vi "test - click.vi"() -> ()   [LabVIEW 2020]
uses:
  <vilib>/Utility/miscctls.llb/LVPositionTypeDef.ctl
  <vilib>/Utility/miscctls.llb/LVPointTypeDef.ctl
  ui-testing.lvlib
  User32.dll
panel:
  out "Screen Coordinates":T1
  out "PanelCoords 2":T1
  out "PanelCoords":T1
  out "Position":T2
  in  "OK Button":bool
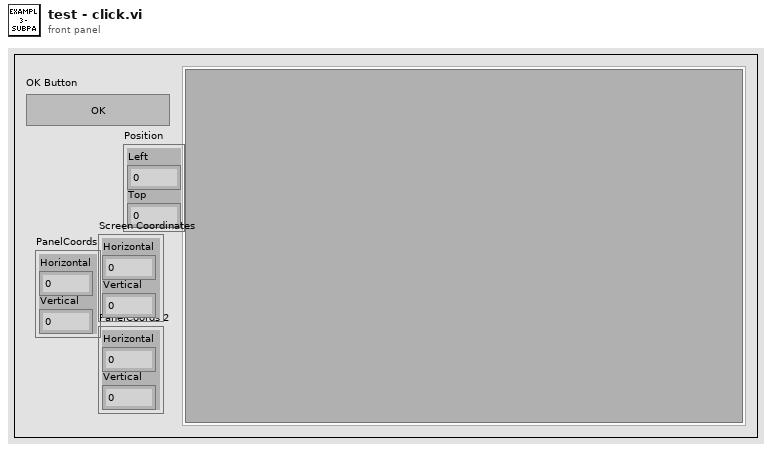
[diagram p1: front panel]
types:
  T1 = typedef "LVPointTypeDef.ctl" = cluster{"Horizontal":i16, "Vertical":i16}
  T2 = typedef "LVPositionTypeDef.ctl" = cluster{"Left":i32, "Top":i32}
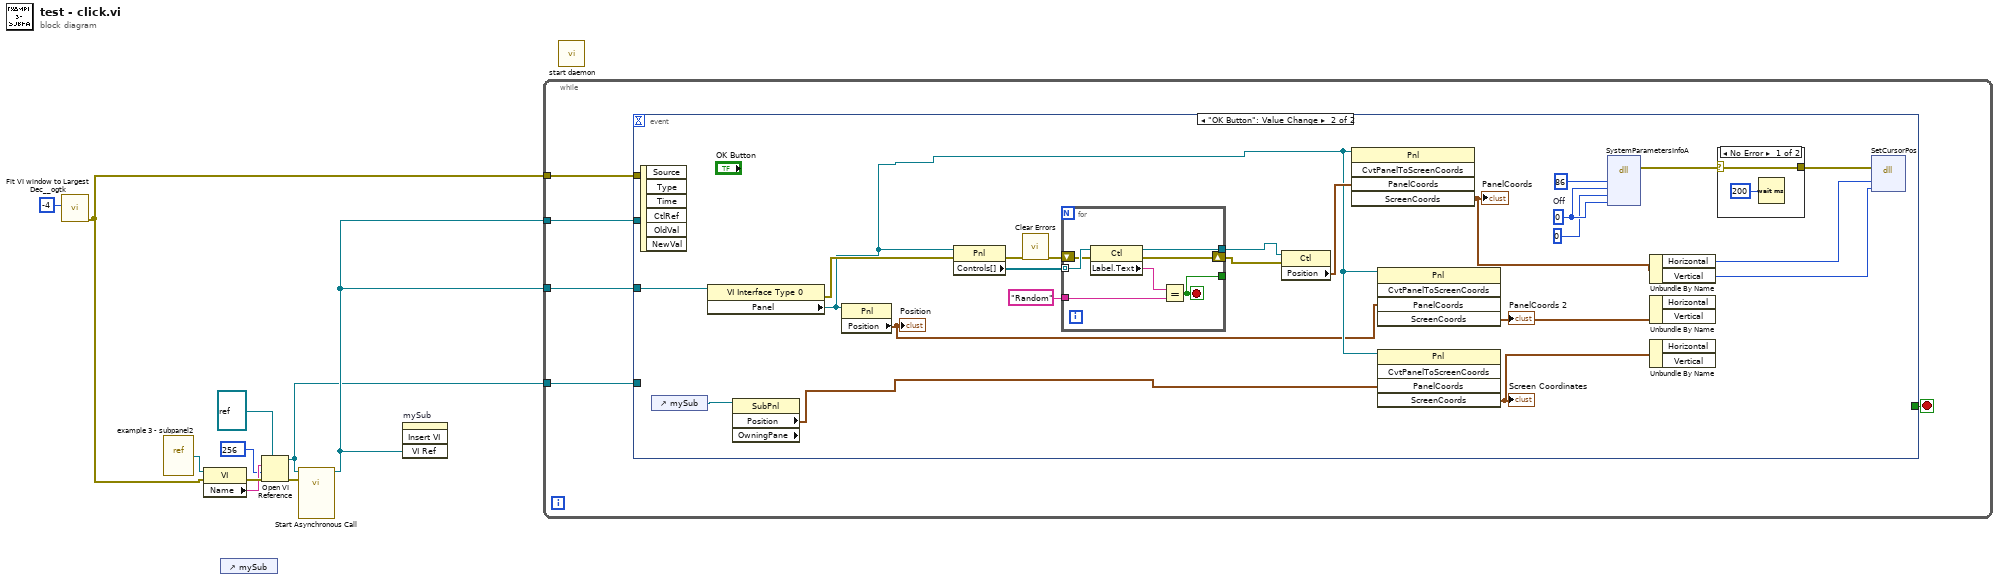
[diagram p0: block diagram]
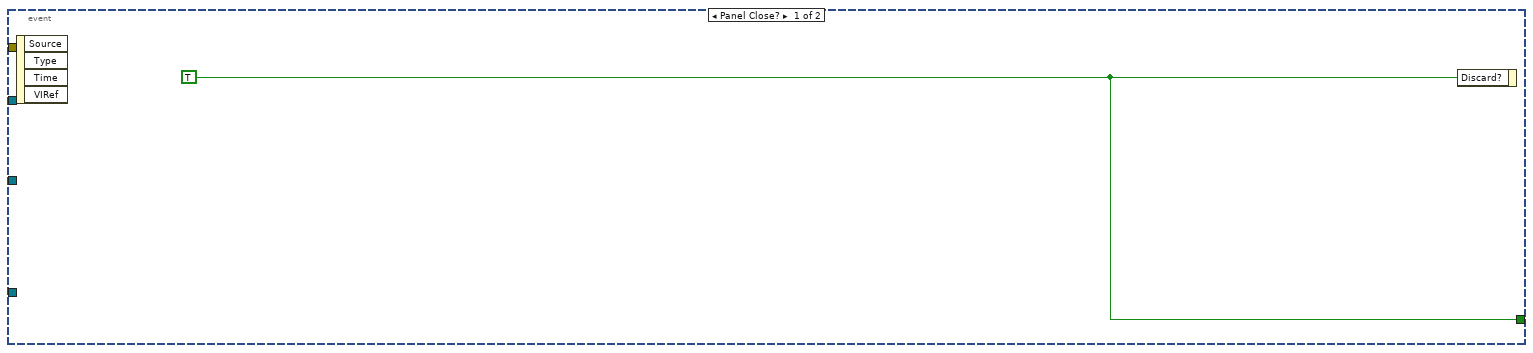
[diagram p2: hidden frame]
diagram:
  n1 = call <userlib>:"Fit VI window to Largest Dec__ogtk.vi"("border spacing (2 px)"=-4) -> ("error out"=w3:errorcluster)  [unwired: 5 in, 1 out]
  n2 = vi-ref "example 3 - subpanel2.vi"() -> (w8:refnum<vi>)
  n3 = property class="VI"(reference=w8, error in=w3) -> (error out=w10:errorcluster, "Name"=w9:string)  [unwired: 1 out]
  n4 = control-ref of="mySub"() -> ()  [unwired: 1 out]
  n5 = Open VI Reference(type specifier VI Refnum (for type only)=refnum<vi> refnum, vi path=w9, options=256 ("call and forget"), error in (no error)=w10) -> (vi reference=w1:refnum<vi>, error out=w7:errorcluster)  [unwired: 2 in]
  n6 = call-by-ref "Start Asynchronous Call"(reference=w1, error in=w7) -> (reference out=w2:refnum<vi>)  [unwired: 12 in, 1 out]
  n7 = invoke on="mySub" class="SubPnl" method="Insert VI"("VI Ref"=w2) -> ()  [unwired: 3 in, 4 out]
  n8 = while {
    tunnel: w3 -> [w14]
    tunnel: w2 -> [w13]
    tunnel: w2 -> [w12]
    tunnel: w1 -> [w11]
    stop <- w15 stop-if-true
    n9 = event shown="[1] \"OK Button\": Value Change" {
      selector: _ -> [_ _]
      dyn-events: _ -> [_ _]
      timeout: _ -> [_ _]
      tunnel: [w16 _] -> w15
      tunnel: w14 -> [_ _]
      tunnel: w13 -> [_ _]
      tunnel: w12 -> [_ w39]
      tunnel: w11 -> [_ _]
      event Panel Close? {
        w16 = TRUE
        n10 = event-data() -> ()  [unwired: 1 in, 4 out]
        n11 = event-data("Discard?"=w16) -> ()  [unwired: 1 in, 1 out]
      }
      event "OK Button": Value Change {
        w26 = u32 0  # Off
        n12 = event-data() -> ()  [unwired: 1 in, 6 out]
        n13 = control-ref of="mySub"() -> (w38:refnum<vi>)
        n14 = property class="VI Interface Type 0"(reference=w39) -> (error out=w34:errorcluster, "Panel"=w29:refnum<vi>)  [unwired: 1 in, 1 out]
        n15 = property class="SubPnl" props=["Position", "OwningPane"](reference=w38) -> ("Position"=w28:T2)  [unwired: 1 in, 3 out]
        n16 = property class="Pnl"(reference=w29) -> ("Position"=w27:T2)  [unwired: 1 in, 2 out]
        "Position" <- w27
        n17 = property class="Pnl"(reference=w29, error in=w34) -> (error out=w36:errorcluster, "Controls[]"=w37:refnum<vi>[])  [unwired: 1 out]
        n18 = call <vilib>:"Clear Errors.vi"("error in (no error)"=w36) -> ("error out"=w35:errorcluster)  [unwired: 5 in, 1 out]
        n19 = for {
          tunnel: w37 -> [w49] mode=indexing
          tunnel: "Random" ("Control Label") -> [w47]
          tunnel: [w46] -> w32
          shift-right: [w44] -> w31
          shift-left: w35 -> [w45]
          tunnel: [w43] -> _
          stop <- w43 stop-if-true
          n20 = property class="Ctl"(reference=w49, error in=w45) -> (reference out=w46:refnum<vi>, error out=w44:errorcluster, "Label.Text"=w48:string)
          n21 = Equal?(x=w48, y=w47) -> (x = y?=w43:bool)
        }
        n22 = property class="Ctl"(reference=w32, error in=w31) -> ("Position"=w30:T2)  [unwired: 2 out]
        n23 = invoke class="Pnl" method="CvtPanelToScreenCoords"(reference=w29, "PanelCoords"=w30) -> ("ScreenCoords"=w21:T1)  [unwired: 3 in, 4 out]
        "PanelCoords" <- w21
        n24 = invoke class="Pnl" method="CvtPanelToScreenCoords"(reference=w29, "PanelCoords"=w27) -> ("ScreenCoords"=w19:T1)  [unwired: 3 in, 4 out]
        "PanelCoords 2" <- w19
        n25 = invoke class="Pnl" method="CvtPanelToScreenCoords"(reference=w29, "PanelCoords"=w28) -> ("ScreenCoords"=w20:T1)  [unwired: 3 in, 4 out]
        "Screen Coordinates" <- w20
        n26 = dll-call lib="User32.dll" fn="SystemParametersInfoA" label="Terminate power-off mode"("uiAction"=u32 86 ("SPI_GETPOWEROFFACTIVE"), "uiParam"=w26, "pvParam"=0, "fWinIni"=w26) -> (error out=w23:errorcluster)  [unwired: 8 in, 1 out]
        n27 = Unbundle By Name(w21) -> ("Horizontal"=w18:i16, "Vertical"=w17:i16)
        n28 = Unbundle By Name(w19) -> ()  [unwired: 2 out]
        n29 = Unbundle By Name(w20) -> ()  [unwired: 2 out]
        n30 = case shown="No Error" w23 {
          selector: w23 -> [w40 w42]
          tunnel: [w40 w42] -> w22
          frame No Error {
            n31 = Wait (ms)(milliseconds to wait=u32 200) -> ()  [unwired: 1 out]
          }
          frame Error {
          }
        }
        n32 = dll-call lib="User32.dll" fn="SetCursorPos" label="Move mouse"(error in=w22, "dx"=w18, "dy"=w17) -> ()  [unwired: 5 in, 2 out]
      }
    }
  }
  n33 = call "start daemon.vi"() -> ()  [unwired: 11 in, 1 out]
